vi "OOK_FrameAnalysis.vi"(11 "input bit stream":i8[](array[numeric])) -> (3 "data bit stream":i8[](array[numeric]))   [LabVIEW 2014]
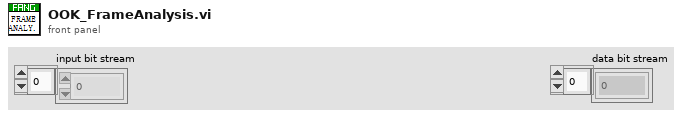
[diagram p1: front panel]
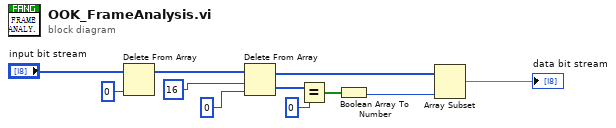
[diagram p0: block diagram]
diagram:
  n1 = Delete From Array(array="input bit stream", index=0) -> (array with subset deleted=w10:i8[])  [unwired: 1 in, 1 out]
  n2 = Delete From Array(array=w10, length=16 ("index"), index=0 ("length")) -> (deleted portion=w6:i8[], array with subset deleted=w3:i8[])
  n3 = Equal?(x=w6, y=i8 0) -> (x = y?=w5:bool[])
  n4 = Boolean Array To Number(Boolean array=w5) -> (number=w2:u32)
  n5 = Array Subset(array=w3, length=w2) -> (→"data bit stream":i8[])  [unwired: 1 in]
